vi "EVT Camera Get String Param.vi"(6 "valueSize":u32, 7 "bufferSize":u32, 9 "buffer":string, 10 "name":string, 11 "camera":u64) -> (1 "buffer out":string, 3 "function return":u32(ring), 4 "valueSize out":u32)   [LabVIEW 2019, in "EmergentCameraC.lvlib"]
doc: "EMERGENTCAMERAC_API EVT_ERROR EVT_CameraGetStringParam(Camera_Handle camera, const char* name, char* buffer, unsigned long bufferSize, unsigned long* valueSize);"
uses:
  EmergentCameraC.lvlib
  emergentInstall_Windows/win64/eSDK/bin/EmergentCameraC.dll
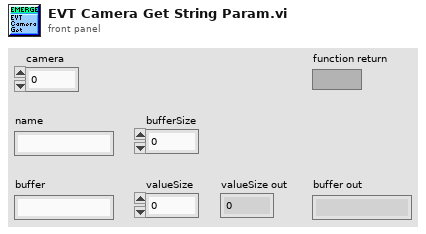
[diagram p1: front panel]
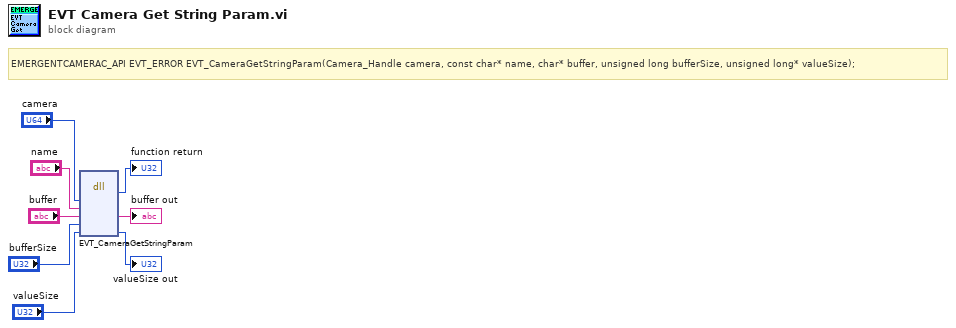
[diagram p0: block diagram]
diagram:
  # "EMERGENTCAMERAC_API EVT_ERROR EVT_CameraGetStringParam(Camera_Handle camera, const char* name, char* buffer, unsigned long bufferSize, unsigned long* valueSize);"
  n1 = dll-call lib="E:/emergent/host-new_QT/emergentInstall_Windows/win64/eSDK/bin/EmergentCameraC.*" fn="EVT_CameraGetStringParam"("camera"="camera", "name"="name", "buffer"="buffer", "bufferSize"="bufferSize", "valueSize"="valueSize") -> (→"function return":u32, "buffer"=→"buffer out":string, "valueSize"=→"valueSize out":u32)  [unwired: 6 in, 2 out]
